vi "(Sub) CMD Parsing_3.vi"(0 "Set V":dbl, 1 "State":T1, 5 "Set mA":dbl, 7 "CMD Get V":string, 9 "CMD Get mA":string, 11 "error in (no error)":errorcluster caption="에러 입력(에러 없음)", 12 "CMD Get ADC":string) -> (4 "CMD Set V":string, 6 "CMD Set mA":string, 8 "Get KV":dbl, 10 "Get mA":dbl, 15 "error out":errorcluster caption="에러 출력")   [LabVIEW 2017]
uses:
  Controls/(Ctrl) State_Parcing.ctl
  <vilib>/regexp/Match Regular Expression.xnode
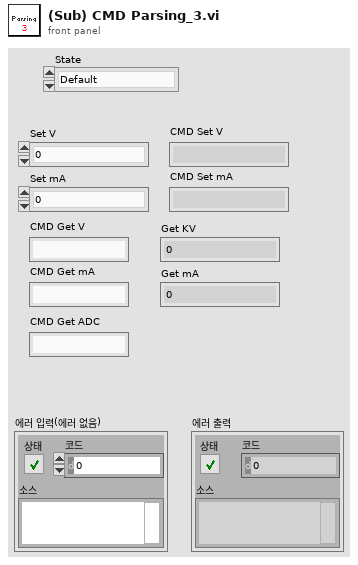
[diagram p1: front panel]
types:
  T1 = typedef "(Ctrl) State_Parcing.ctl" = enum16{"Default", "Set V", "Set mA", "Get V", "Get mA", "Get ADC"}
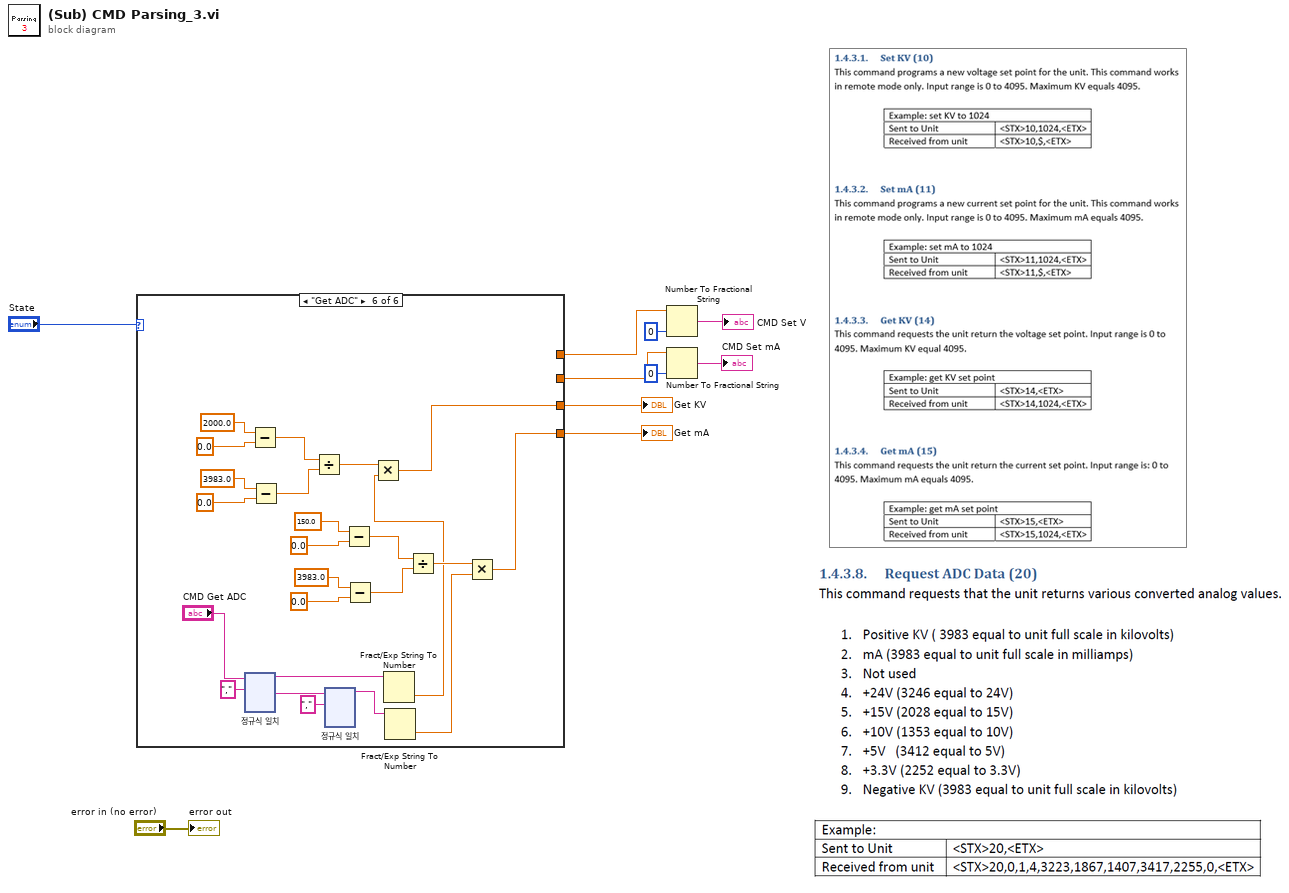
[diagram p0: block diagram]
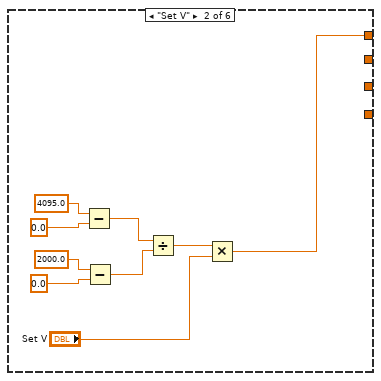
[diagram p3: hidden frame]
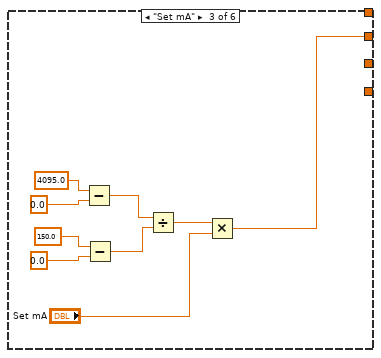
[diagram p4: hidden frame]
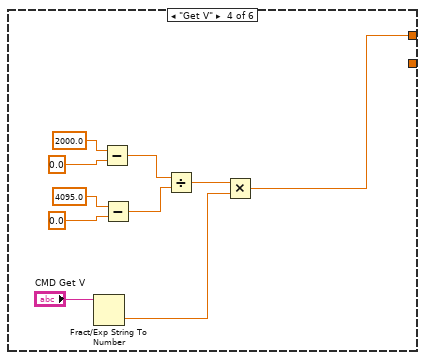
[diagram p5: hidden frame]
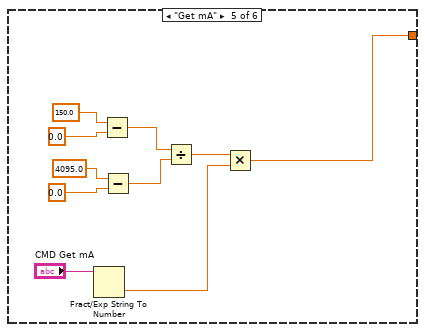
[diagram p6: hidden frame]
diagram:
  n1 = case shown="\"Get ADC\"" "State" {
    tunnel: [_ w11 _ _ _ _] -> w6
    tunnel: [_ _ w20 _ _ _] -> w5
    tunnel: [_ _ _ w29 _ w51] -> w8
    tunnel: [_ _ _ _ w39 w50] -> w7
    frame "Default", Default {
    }
    frame "Set V" {
      n2 = Subtract(x=4095.0, y=0.0) -> (x-y=w17:dbl)
      n3 = Subtract(x=2000.0, y=0.0) -> (x-y=w18:dbl)
      n4 = Divide(x=w17, y=w18) -> (x/y=w19:dbl)
      n5 = Multiply(x=w19, y="Set V") -> (x*y=w11:dbl)
    }
    frame "Set mA" {
      n6 = Subtract(x=4095.0, y=0.0) -> (x-y=w26:dbl)
      n7 = Subtract(x=150.0, y=0.0) -> (x-y=w27:dbl)
      n8 = Divide(x=w26, y=w27) -> (x/y=w28:dbl)
      n9 = Multiply(x=w28, y="Set mA") -> (x*y=w20:dbl)
    }
    frame "Get V" {
      n10 = Fract/Exp String To Number(string="CMD Get V") -> (number=w30:dbl)  [unwired: 3 in, 1 out]
      n11 = Subtract(x=2000.0, y=0.0) -> (x-y=w35:dbl)
      n12 = Subtract(x=4095.0, y=0.0) -> (x-y=w36:dbl)
      n13 = Divide(x=w35, y=w36) -> (x/y=w37:dbl)
      n14 = Multiply(x=w37, y=w30) -> (x*y=w29:dbl)
    }
    frame "Get mA" {
      n15 = Fract/Exp String To Number(string="CMD Get mA") -> (number=w40:dbl)  [unwired: 3 in, 1 out]
      n16 = Subtract(x=150.0, y=0.0) -> (x-y=w45:dbl)
      n17 = Subtract(x=4095.0, y=0.0) -> (x-y=w46:dbl)
      n18 = Divide(x=w45, y=w46) -> (x/y=w47:dbl)
      n19 = Multiply(x=w47, y=w40) -> (x*y=w39:dbl)
    }
    frame "Get ADC" {
      n20 = xnode "정규식 일치"("입력 문자열"="CMD Get ADC", "정규식"=",") -> ("일치 구문 앞"=w61:string, "일치 구문 뒤"=w62:string)  [unwired: 4 in, 3 out]
      n21 = Subtract(x=2000.0, y=0.0) -> (x-y=w70:dbl)
      n22 = Subtract(x=3983.0, y=0.0) -> (x-y=w71:dbl)
      n23 = Divide(x=w70, y=w71) -> (x/y=w72:dbl)
      n24 = xnode "정규식 일치"("입력 문자열"=w62, "정규식"=",") -> ("일치 구문 앞"=w60:string)  [unwired: 4 in, 4 out]
      n25 = Subtract(x=150.0, y=0.0) -> (x-y=w55:dbl)
      n26 = Subtract(x=3983.0, y=0.0) -> (x-y=w54:dbl)
      n27 = Fract/Exp String To Number(string=w61) -> (number=w49:dbl)  [unwired: 3 in, 1 out]
      n28 = Multiply(x=w72, y=w49) -> (x*y=w51:dbl)
      n29 = Fract/Exp String To Number(string=w60) -> (number=w52:dbl)  [unwired: 3 in, 1 out]
      n30 = Divide(x=w55, y=w54) -> (x/y=w53:dbl)
      n31 = Multiply(x=w53, y=w52) -> (x*y=w50:dbl)
    }
  }
  "Get KV" <- w8
  "Get mA" <- w7
  n32 = Number To Fractional String(number=w6, precision (6)=i16 0 ("정밀도(6)")) -> (F-format string=→"CMD Set V":string)  [unwired: 2 in]
  n33 = Number To Fractional String(number=w5, precision (6)=i16 0 ("정밀도(6)")) -> (F-format string=→"CMD Set mA":string)  [unwired: 2 in]
  "error out" <- "error in (no error)"
